vi "laba5.vi"() -> ()   [LabVIEW 2021]
panel:
  out "?":bool
  out "?":bool
  out "?":bool
  out "?":bool
  out "?":bool
  out "?":bool
  out "?":bool
  in  "min":dbl
  in  "max":dbl
  out "kod":dbl
  out "?":bool
  out "?":bool
  out "?":bool
  out "?":bool
  out "?":bool
  out "?":bool
  out "?":bool
  in  "napr9zhenie":dbl(slide) scale=-10.0..10.0
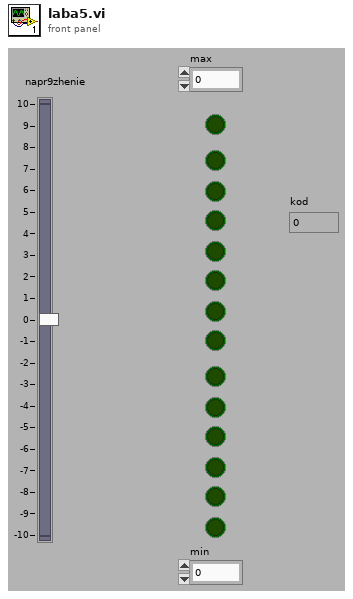
[diagram p1: front panel]
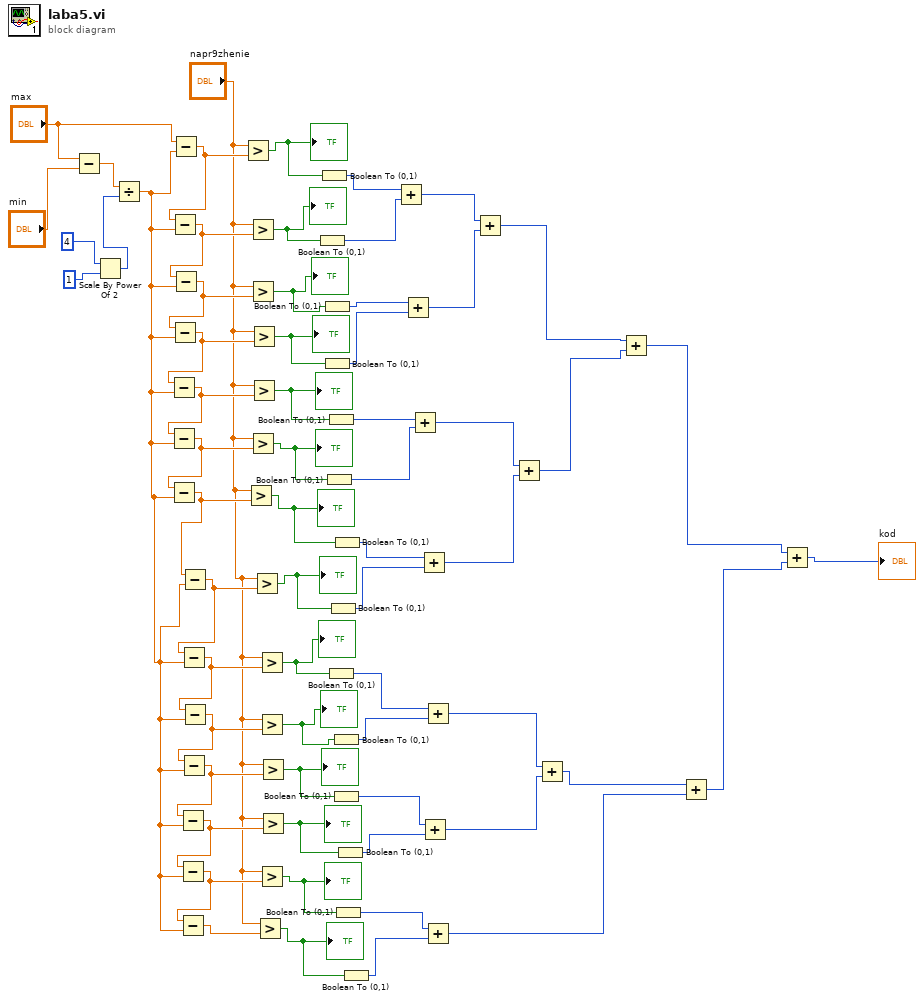
[diagram p0: block diagram]
diagram:
  n1 = Subtract(x="max", y="min") -> (x-y=w37:dbl)
  n2 = Scale By Power Of 2(n=4, x=1) -> (x*2^n=w38:i32)
  n3 = Divide(x=w37, y=w38) -> (x/y=w21:dbl)
  n4 = Subtract(x="max", y=w21) -> (x-y=w59:dbl)
  n5 = Subtract(x=w59, y=w21) -> (x-y=w60:dbl)
  n6 = Subtract(x=w60, y=w21) -> (x-y=w61:dbl)
  n7 = Subtract(x=w61, y=w21) -> (x-y=w58:dbl)
  n8 = Subtract(x=w58, y=w21) -> (x-y=w57:dbl)
  n9 = Subtract(x=w57, y=w21) -> (x-y=w56:dbl)
  n10 = Subtract(x=w56, y=w21) -> (x-y=w22:dbl)
  n11 = Subtract(x=w22, y=w21) -> (x-y=w33:dbl)
  n12 = Subtract(x=w33, y=w21) -> (x-y=w34:dbl)
  n13 = Subtract(x=w34, y=w21) -> (x-y=w35:dbl)
  n14 = Subtract(x=w35, y=w21) -> (x-y=w32:dbl)
  n15 = Subtract(x=w32, y=w21) -> (x-y=w31:dbl)
  n16 = Subtract(x=w31, y=w21) -> (x-y=w30:dbl)
  n17 = Subtract(x=w30, y=w21) -> (x-y=w36:dbl)
  n18 = Greater?(x="napr9zhenie", y=w59) -> (0:w49:bool)
  "?" <- w49
  n19 = Greater?(x="napr9zhenie", y=w22) -> (0:w55:bool)
  "?" <- w55
  n20 = Greater?(x="napr9zhenie", y=w60) -> (0:w50:bool)
  "?" <- w50
  n21 = Greater?(x="napr9zhenie", y=w61) -> (0:w51:bool)
  "?" <- w51
  n22 = Greater?(x="napr9zhenie", y=w56) -> (0:w54:bool)
  "?" <- w54
  n23 = Greater?(x="napr9zhenie", y=w58) -> (0:w52:bool)
  "?" <- w52
  n24 = Greater?(x="napr9zhenie", y=w57) -> (0:w53:bool)
  "?" <- w53
  n25 = Greater?(x="napr9zhenie", y=w33) -> (0:w23:bool)
  "?" <- w23
  n26 = Greater?(x="napr9zhenie", y=w36) -> (0:w29:bool)
  "?" <- w29
  n27 = Greater?(x="napr9zhenie", y=w34) -> (0:w24:bool)
  "?" <- w24
  n28 = Greater?(x="napr9zhenie", y=w35) -> (0:w25:bool)
  "?" <- w25
  n29 = Greater?(x="napr9zhenie", y=w30) -> (0:w28:bool)
  "?" <- w28
  n30 = Greater?(x="napr9zhenie", y=w32) -> (0:w26:bool)
  "?" <- w26
  n31 = Greater?(x="napr9zhenie", y=w31) -> (0:w27:bool)
  "?" <- w27
  n32 = Boolean To (0,1)(Boolean=w50) -> (0, 1=w47:i16)
  n33 = Boolean To (0,1)(Boolean=w49) -> (0, 1=w48:i16)
  n34 = Boolean To (0,1)(Boolean=w51) -> (0, 1=w46:i16)
  n35 = Boolean To (0,1)(Boolean=w52) -> (0, 1=w45:i16)
  n36 = Boolean To (0,1)(Boolean=w54) -> (0, 1=w43:i16)
  n37 = Boolean To (0,1)(Boolean=w53) -> (0, 1=w44:i16)
  n38 = Boolean To (0,1)(Boolean=w24) -> (0, 1=w17:i16)
  n39 = Boolean To (0,1)(Boolean=w23) -> (0, 1=w18:i16)
  n40 = Boolean To (0,1)(Boolean=w25) -> (0, 1=w16:i16)
  n41 = Boolean To (0,1)(Boolean=w26) -> (0, 1=w15:i16)
  n42 = Boolean To (0,1)(Boolean=w55) -> (0, 1=w19:i16)
  n43 = Boolean To (0,1)(Boolean=w28) -> (0, 1=w13:i16)
  n44 = Boolean To (0,1)(Boolean=w27) -> (0, 1=w14:i16)
  n45 = Boolean To (0,1)(Boolean=w29) -> (0, 1=w12:i16)
  n46 = Add(x=w48, y=w47) -> (x+y=w41:i16)
  n47 = Add(x=w46, y=w45) -> (x+y=w42:i16)
  n48 = Add(x=w44, y=w43) -> (x+y=w11:i16)
  n49 = Add(x=w19, y=w18) -> (x+y=w10:i16)
  n50 = Add(x=w15, y=w14) -> (x+y=w8:i16)
  n51 = Add(x=w17, y=w16) -> (x+y=w9:i16)
  n52 = Add(x=w13, y=w12) -> (x+y=w7:i16)
  n53 = Add(x=w41, y=w42) -> (x+y=w5:i16)
  n54 = Add(x=w11, y=w10) -> (x+y=w4:i16)
  n55 = Add(x=w9, y=w8) -> (x+y=w6:i16)
  n56 = Add(x=w5, y=w4) -> (x+y=w3:i16)
  n57 = Add(x=w6, y=w7) -> (x+y=w2:i16)
  n58 = Add(x=w3, y=w2) -> (x+y=→"kod":i16)
